vi "FormatString.vi"(8 "Error In":errorcluster, 11 "Input string":string) -> (0 "Error Out":errorcluster, 3 "resulting string":string)   [LabVIEW 2018]
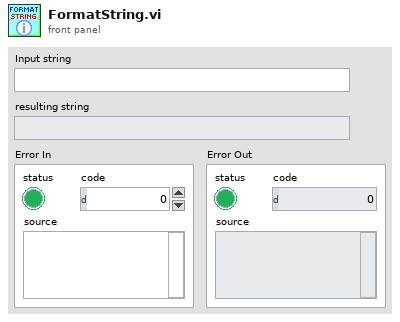
[diagram p1: front panel]
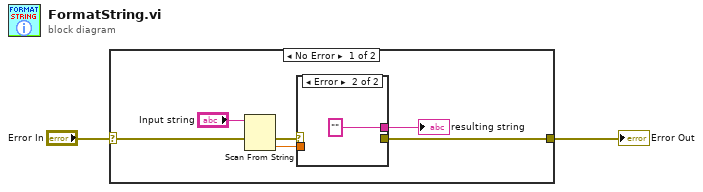
[diagram p0: block diagram]
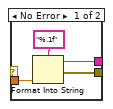
[diagram p2: hidden frame]
diagram:
  n1 = case shown="No Error" "Error In" {
    selector: "Error In" -> [w7 w14]
    tunnel: [w3 w14] -> w1
    frame No Error {
      n2 = Scan From String(input string="Input string", error in=w7) -> (error out=w5:errorcluster, output 1=w6:dbl)  [unwired: 3 in, 2 out]
      n3 = case shown="Error" w5 {
        tunnel: w6 -> [w11 _]
        tunnel: [w10 ""] -> w4
        tunnel: [w9 _] -> w3
        frame No Error {
          n4 = Format Into String(format string="%.1f", w11) -> (resulting string=w10:string, error out=w9:errorcluster)  [unwired: 2 in]
        }
        frame Error {
        }
      }
      "resulting string" <- w4
    }
    frame Error {
    }
  }
  "Error Out" <- w1
